vi "determine COM baud rate.vi"(11 "VISA resource name":refnum<visa-resource-name>="COM3") -> (0 "error out":errorcluster, 1 "Stage found?":bool, 2 "card type (F for old cards, T for new cards)":bool, 3 "VISA resource name out":refnum<visa-resource-name>)   [LabVIEW 2012]
doc: "SciScan 1.2 160622"
uses:
  <vilib>/Instr/_visa.llb/VISA Configure Serial Port (Instr).vi
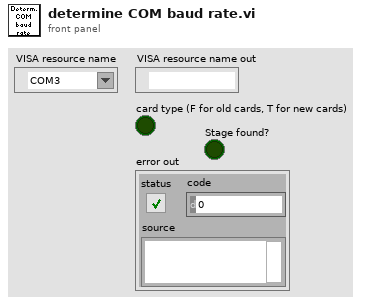
[diagram p1: front panel]
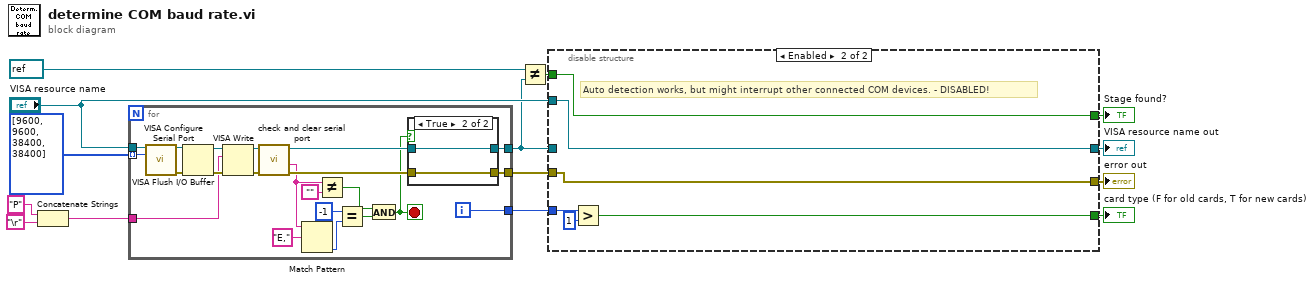
[diagram p0: block diagram]
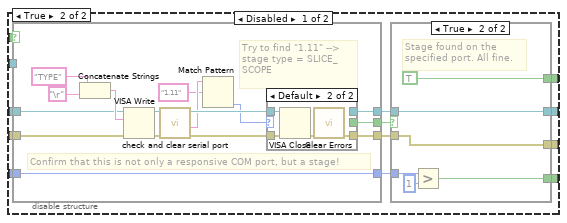
[diagram p2: hidden frame]
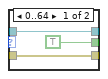
[diagram p4: hidden frame]
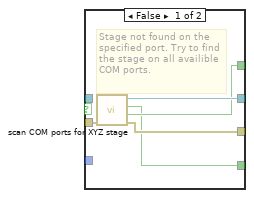
[diagram p5: hidden frame]
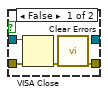
[diagram p6: hidden frame]
diagram:
  n1 = Concatenate Strings("P" ("write buffer"), "\r") -> (w10:string)
  n2 = for {
    tunnel: u32[] [9600, 9600, 38400, 38400] -> [w19] mode=indexing
    tunnel: [w20] -> w3
    tunnel: "VISA resource name" -> [w18]
    tunnel: w10 -> [w17]
    tunnel: [w16] -> w5
    tunnel: [w15] -> w1
    i -> [w20]
    stop <- w21 stop-if-true
    n3 = call-poly "VISA Configure Serial Port"("VISA resource name"=w18, "baud rate (9600)"=w19) -> ("VISA resource name out"=w35:refnum<visa-resource-name>, "error out"=w36:errorcluster)  [unwired: 12 in]
    n4 = VISA Flush I/O Buffer(VISA resource name=w35, error in (no error)=w36) -> (VISA resource name out=w32:refnum<visa-resource-name>, error out=w31:errorcluster)  [unwired: 1 in]
    n5 = VISA Write(VISA resource name=w32, write buffer=w17, error in (no error)=w31) -> (VISA resource name out=w34:refnum<visa-resource-name>, error out=w33:errorcluster)  [unwired: 1 out]
    n6 = call "check and clear serial port.vi"("error in (no error)"=w33, "VISA resource name in"=w34) -> ("error out"=w29:errorcluster, "read buffer"=w27:string, "VISA resource name out"=w30:refnum<visa-resource-name>)  [unwired: 6 in, 1 out]
    n7 = Match Pattern(string=w27, regular expression="E,") -> (offset past match=w25:i32)  [unwired: 1 in, 3 out]
    n8 = Not Equal?(x=w27, y="") -> (x != y?=w23:bool)
    n9 = Equal?(x=-1, y=w25) -> (x = y?=w22:bool)
    n10 = And(x=w23, y=w22) -> (x .and. y?=w21:bool)
    n11 = case shown="True" w21 {
      tunnel: w30 -> [w40 w41]
      tunnel: w29 -> [w39 w42]
      tunnel: [w37 w42] -> w16
      tunnel: [_ w41] -> w15
      frame False {
        n12 = VISA Close(VISA resource name=w40, error in (no error)=w39) -> (error out=w38:errorcluster)
        n13 = call <vilib>:"Clear Errors.vi"("error in (no error)"=w38) -> ("error out"=w37:errorcluster)  [unwired: 6 in]
      }
      frame True {
      }
    }
  }
  n14 = Not Equal?(x=refnum<visa-resource-name> refnum ("VISA resource name out"), y=w1) -> (x != y?=w4:bool)
  n15 = disable-structure shown="Enabled" {
    disable-tunnel: [w54 w95] -> w13
    disable-tunnel: [w53 w93] -> w8
    disable-tunnel: [w52 w98] -> w7
    disable-tunnel: [w51 w94] -> w6
    disable-tunnel: w5 -> [w50 w98]
    disable-tunnel: w1 -> [w47 _]
    disable-tunnel: w4 -> [w46 w94]
    disable-tunnel: w3 -> [w45 w96]
    disable-tunnel: "VISA resource name" -> [_ w93]
    frame Disabled {
      n16 = case shown="True" w46 {
        selector: w46 -> [w55 _]
        tunnel: w50 -> [w58 w71]
        tunnel: [w58 w63] -> w49
        tunnel: [w57 w62] -> w48
        tunnel: w47 -> [w57 w61]
        tunnel: w45 -> [w56 w60]
        tunnel: [w56 w60] -> w44
        tunnel: [w55 w59] -> w43
        frame False {
        }
        frame True {
          # "Try to find \"1.11\" --> stage type = SLICE_SCOPE"
          # "Confirm that this is not only a responsive COM port, but a stage!"
          n17 = Concatenate Strings("TYPE" ("write buffer"), "\r") -> (w74:string)
          n18 = VISA Write(VISA resource name=w61, write buffer=w74, error in (no error)=w71) -> (VISA resource name out=w65:refnum<visa-resource-name>, error out=w64:errorcluster)  [unwired: 1 out]
          n19 = call "check and clear serial port.vi"("error in (no error)"=w64, "VISA resource name in"=w65) -> ("error out"=w69:errorcluster, "read buffer"=w67:string, "VISA resource name out"=w70:refnum<visa-resource-name>)  [unwired: 6 in, 1 out]
          n20 = Match Pattern(string=w67, regular expression="1.11" ("read buffer")) -> (offset past match=w68:i32)  [unwired: 1 in, 3 out]
          n21 = case shown="Default" w68 {
            tunnel: w70 -> [w76 w81]
            tunnel: w69 -> [w77 w80]
            tunnel: [w77 w78] -> w63
            tunnel: [w76 _] -> w62
            tunnel: [TRUE _] -> w59
            frame 0..64 {
            }
            frame Default {
              n22 = VISA Close(VISA resource name=w81, error in (no error)=w80) -> (error out=w79:errorcluster)
              n23 = call <vilib>:"Clear Errors.vi"("error in (no error)"=w79) -> ("error out"=w78:errorcluster)  [unwired: 6 in]
            }
          }
        }
      }
      n24 = case shown="True" w43 {
        tunnel: w44 -> [_ w92]
        tunnel: [w82 w90] -> w54
        tunnel: w48 -> [_ w88]
        tunnel: [w85 w88] -> w53
        tunnel: w49 -> [w86 w87]
        tunnel: [w84 w87] -> w52
        tunnel: [w83 TRUE ("Stage found?")] -> w51
        frame False {
          # "Stage not found on the specified port. Try to find the stage on all availible COM ports."
          n25 = call "scan COM ports for XYZ stage.vi"("error in (no error)"=w86) -> ("error out"=w84:errorcluster, "Stage found?"=w83:bool, "card type (F for old cards, T for new cards)"=w82:bool, "VISA resource name out"=w85:refnum<visa-resource-name>)  [unwired: 7 in]
        }
        frame True {
          # "Stage found on the specified port. All fine."
          n26 = Greater?(x=w92, y=1) -> (0:w90:bool)
        }
      }
    }
    frame Enabled {
      # "Auto detection works, but might interrupt other connected COM devices. - DISABLED!"
      n27 = Greater?(x=w96, y=1) -> (0:w95:bool)
    }
  }
  "card type (F for old cards, T for new cards)" <- w13
  "VISA resource name out" <- w8
  "error out" <- w7
  "Stage found?" <- w6
